vi "Create FIFO Config.vi"(11 "New FIFO Config":T1) -> (3 "Flattened FIFO Config":u8[](array[numeric]))   [LabVIEW 2021, in "ChannelCommon.lvlib"]
doc: "This will create the flattened FIFO configuration used to override the default settings when creating a new FIFO reader or writer. If no configuration is provided the default for that FIFO type will be used. \n\nThis configuration is also used on tag writers with variable length input such as string tags. For tags only the Max Bytes/Msg element is used and other fields are ignored. \n\nIf additional custom data is needed by the FIFO type this can be appended to the end of the flattened data. This custom data will be FIFO specific and is not commonly used."
uses:
  ChannelCommon.lvlib
  typedef/New FIFO Config.ctl
  typedef/FIFO Flags.ctl
  typedef/FIFO Config.ctl
  <vilib>/CIF Foundation/CIF Utilities/DataTypes/Flatten Unflatten/Flatten U64.vi
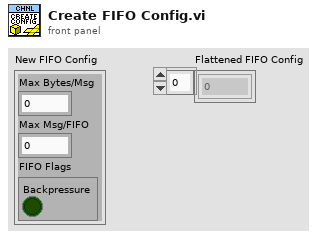
[diagram p1: front panel]
types:
  T1 = typedef "ChannelCommon.lvlib/New FIFO Config.ctl" = cluster{"Max Bytes/Msg":u64, "Max Msg/FIFO":u64, "FIFO Flags":T2}
  T2 = typedef "ChannelCommon.lvlib/FIFO Flags.ctl" = cluster{"Backpressure":bool}
  T3 = typedef "ChannelCommon.lvlib/FIFO Config.ctl" = cluster{"Max Bytes/Msg":u64, "Max Msg/FIFO":u64, "Flags":u64, "Custom Data":u8[]}
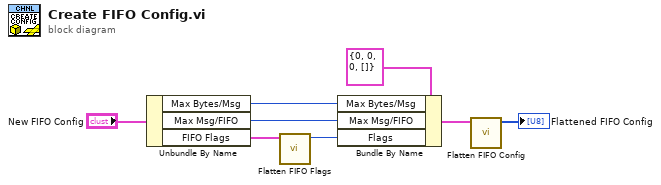
[diagram p0: block diagram]
diagram:
  n1 = Unbundle By Name("New FIFO Config") -> ("Max Bytes/Msg"=w6:u64, "Max Msg/FIFO"=w3:u64, "FIFO Flags"=w5:T2)
  n2 = call "Flatten FIFO Flags.vi"("Flags"=w5) -> ("FIFO Flags"=w4:u64)  [unwired: 10 in]
  n3 = Bundle By Name(cluster=T3 {"Max Bytes/Msg"=0, "Max Msg/FIFO"=0, "Flags"=0, "Custom Data"=[]} ("FIFO Config in"), "Max Bytes/Msg"=w6, "Max Msg/FIFO"=w3, "Flags"=w4) -> (w2:T3)
  n4 = call "Flatten FIFO Config.vi"("FIFO Config in"=w2) -> ("Flattened FIFO Config"=→"Flattened FIFO Config":u8[])  [unwired: 10 in]
